vi "searchInXMLNodes.vi"(8 "error in (no error)":errorcluster, 9 "searchElementName":string, 10 "searchElementIn":string, 11 "xmlNode in":refnum<class "xmlNode.lvclass">) -> (0 "error out":errorcluster, 1 "arrayXmlNodes":refnum<class "xmlNode.lvclass">[](array[class]), 3 "xmlNode out":refnum<class "xmlNode.lvclass">)   [LabVIEW 2009, in "Tools.lvlib" / "xml.lvlib" / "xmlNode.lvclass"]
uses:
  xmlNode.lvclass
  XmlParser.lvclass
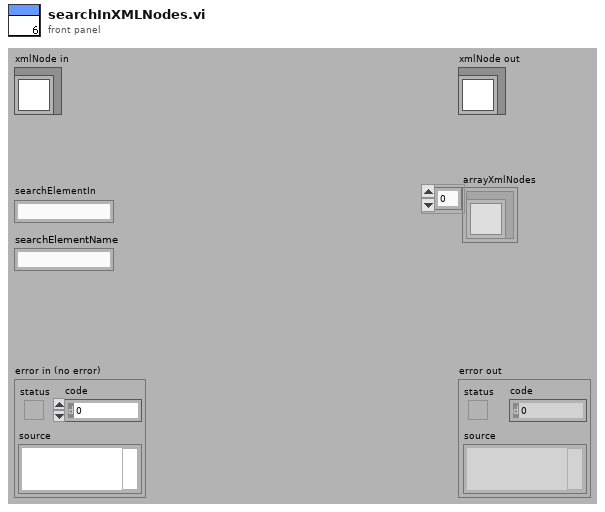
[diagram p1: front panel]
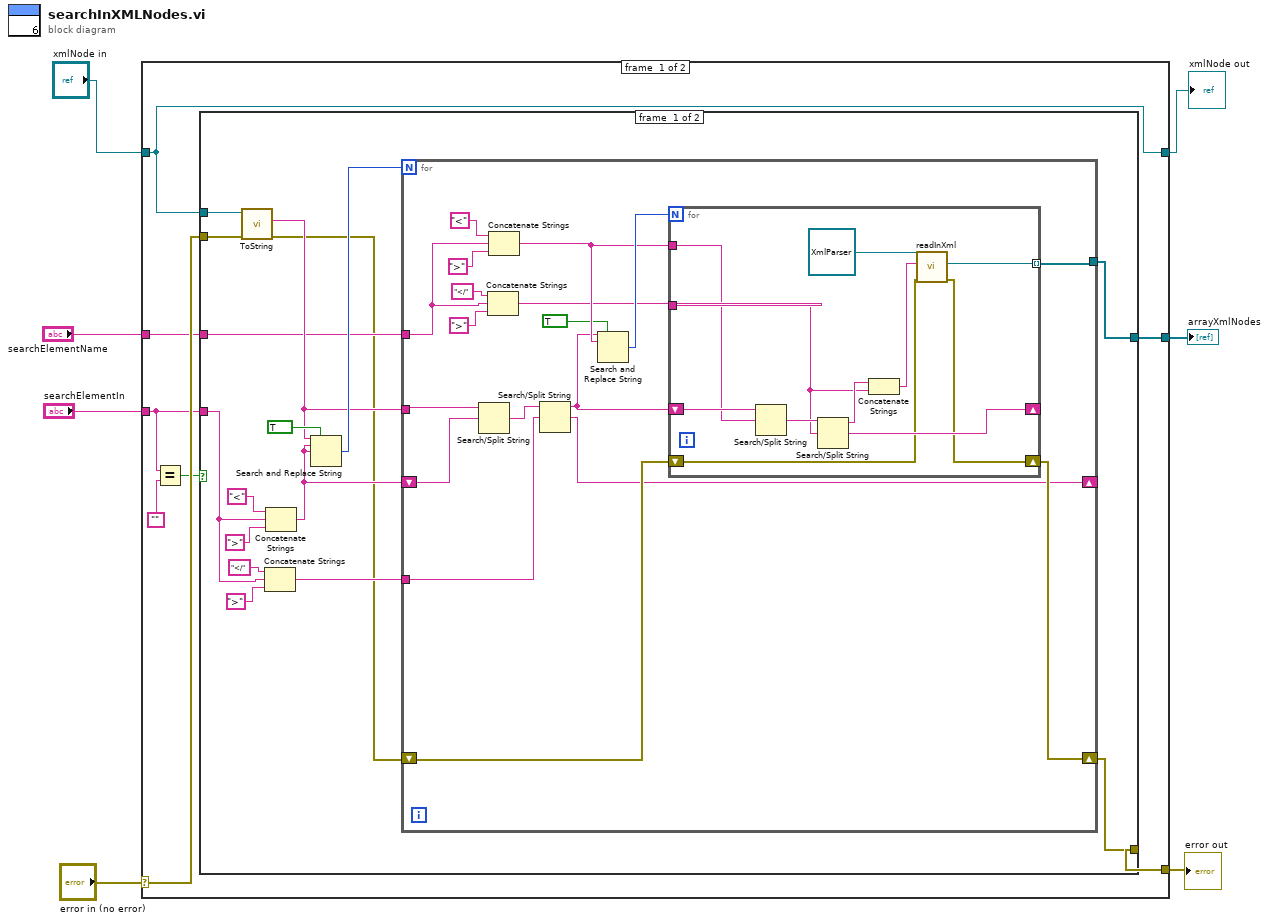
[diagram p0: block diagram]
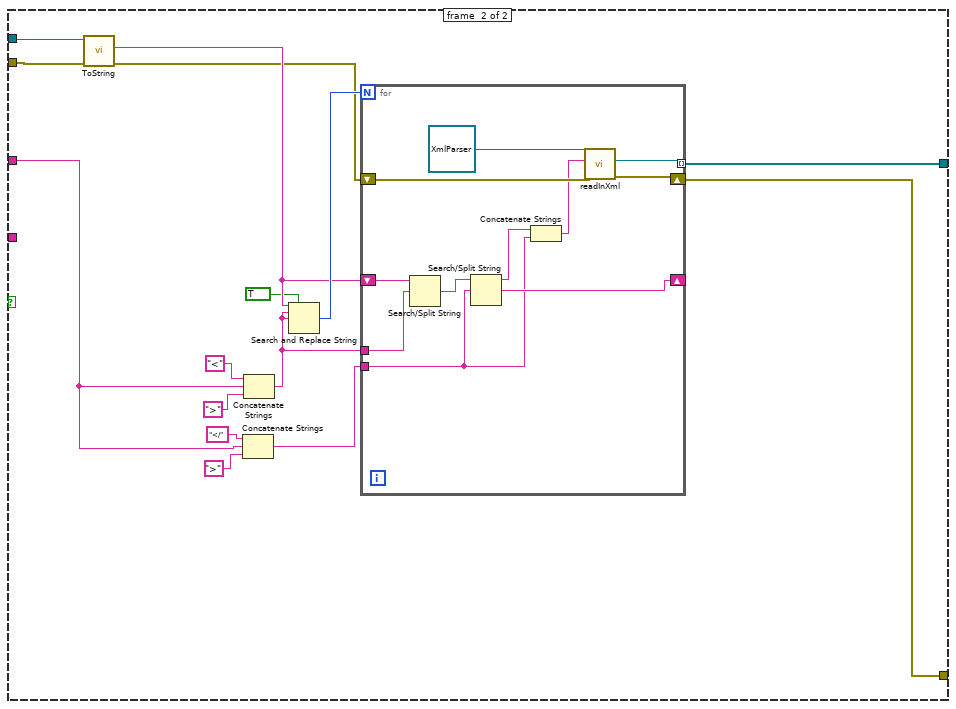
[diagram p2: hidden frame]
diagram:
  n1 = case shown="No Error" "error in (no error)" {
    selector: "error in (no error)" -> [w15 w88]
    tunnel: [w12 w88] -> w6
    tunnel: [w13 w87] -> w4
    tunnel: "xmlNode in" -> [w13 w87]
    tunnel: "searchElementName" -> [w14 _]
    tunnel: "searchElementIn" -> [w9 _]
    tunnel: [w8 _] -> w1
    frame #0 {
      n2 = Equal?(x=w9, y="") -> (x = y?=w11:bool)
      n3 = case shown="False" w11 {
        tunnel: w15 -> [w26 w64]
        tunnel: w9 -> [w25 _]
        tunnel: w14 -> [w20 w63]
        tunnel: w13 -> [w18 w65]
        tunnel: [w17 w62] -> w12
        tunnel: [w16 w61] -> w8
        frame #0 {
          n4 = call-dynamic "ToString.vi"("error in (no error)"=w26, "xmlNode in"=w18) -> ("error out"=w19:errorcluster, "xml"=w23:string)  [unwired: 7 in, 1 out]
          n5 = Concatenate Strings("</", w25, ">") -> (w21:string)
          n6 = Concatenate Strings("<", w25, ">") -> (w22:string)
          n7 = Search and Replace String(replace all?=TRUE, input string=w23, search string=w22, replace string=w22) -> (number of replacements=w24:i32)  [unwired: 4 in, 3 out]
          n8 = for {
            N: w24 -> [_]
            tunnel: w23 -> [w48]
            tunnel: w21 -> [w46]
            tunnel: w20 -> [w41]
            shift-right: [w35] -> w17
            shift-left: w19 -> [w36]
            shift-right: [w33] -> _
            shift-left: w22 -> [w47]
            tunnel: [w32] -> w16
            n9 = Search/Split String(string=w48, search string/char (-)=w47) -> (match + rest of string=w49:string)  [unwired: 1 in, 2 out]
            n10 = Concatenate Strings("</", w41, ">") -> (w38:string)
            n11 = Concatenate Strings("<", w41, ">") -> (w39:string)
            n12 = Search/Split String(string=w49, search string/char (-)=w46) -> (substring before match=w37:string, match + rest of string=w33:string)  [unwired: 1 in, 1 out]
            n13 = Search and Replace String(replace all?=TRUE, input string=w37, search string=w39) -> (number of replacements=w40:i32)  [unwired: 5 in, 3 out]
            n14 = for {
              N: w40 -> [_]
              tunnel: w39 -> [w58]
              tunnel: w38 -> [w56]
              shift-right: [w55] -> _
              shift-left: w37 -> [w59]
              shift-right: [w51] -> w35
              shift-left: w36 -> [w52]
              tunnel: [w50] -> w32 mode=indexing
              n15 = Search/Split String(string=w59, search string/char (-)=w58) -> (match + rest of string=w60:string)  [unwired: 1 in, 2 out]
              n16 = Search/Split String(string=w60, search string/char (-)=w56) -> (substring before match=w57:string, match + rest of string=w55:string)  [unwired: 1 in, 1 out]
              n17 = Concatenate Strings(w57, w56) -> (w53:string)
              n18 = call "readInXml.vi"("error in (no error)"=w52, "xmlString"=w53, "XmlParser in"=refnum<class "XmlParser.lvclass"> refnum ("Tools.lvlib:XmlParser.lvclass")) -> ("error out"=w51:errorcluster, "xmlNode"=w50:refnum<class "xmlNode.lvclass">)  [unwired: 6 in, 1 out]
            }
          }
        }
        frame #1 {
          n19 = call-dynamic "ToString.vi"("error in (no error)"=w64, "xmlNode in"=w65) -> ("error out"=w66:errorcluster, "xml"=w70:string)  [unwired: 7 in, 1 out]
          n20 = Concatenate Strings("</", w63, ">") -> (w67:string)
          n21 = Concatenate Strings("<", w63, ">") -> (w68:string)
          n22 = Search and Replace String(replace all?=TRUE, input string=w70, search string=w68, replace string=w68) -> (number of replacements=w71:i32)  [unwired: 4 in, 3 out]
          n23 = for {
            N: w71 -> [_]
            tunnel: w68 -> [w83]
            shift-right: [w82] -> _
            shift-left: w70 -> [w84]
            tunnel: w67 -> [w81]
            tunnel: [w77] -> w61 mode=indexing
            shift-right: [w76] -> w62
            shift-left: w66 -> [w79]
            n24 = Search/Split String(string=w84, search string/char (-)=w83) -> (match + rest of string=w86:string)  [unwired: 1 in, 2 out]
            n25 = Search/Split String(string=w86, search string/char (-)=w81) -> (substring before match=w85:string, match + rest of string=w82:string)  [unwired: 1 in, 1 out]
            n26 = Concatenate Strings(w85, w81) -> (w78:string)
            n27 = call "readInXml.vi"("error in (no error)"=w79, "xmlString"=w78, "XmlParser in"=refnum<class "XmlParser.lvclass"> refnum ("Tools.lvlib:XmlParser.lvclass")) -> ("error out"=w76:errorcluster, "xmlNode"=w77:refnum<class "xmlNode.lvclass">)  [unwired: 6 in, 1 out]
          }
        }
      }
    }
    frame #1 {
    }
  }
  "error out" <- w6
  "xmlNode out" <- w4
  "arrayXmlNodes" <- w1
